vi "5_SPA_KEYSIGHT_rabi_measurements_(SPA_Aver_Mult_traces-Rabi).vi"() -> ()   [LabVIEW 2013]
uses:
  <vilib>/Analysis/baseanly.llb/Mean (DBL).vi
  <vilib>/Analysis/NI_AALBase.lvlib
panel:
  out "x/y":dbl
  out "Normalised":dbl[][](graph)
  out "(Current)":i32=103
  in  "Program to run":u16(ring) items=["Rabi", "T2"]
  in  "?":enum32{"VNA", "SPA"}(tab)
  in  "Center Freq (Hz)":dbl=6953330000.0 caption="Center Freq (Hz):" format="%#.6p"
  in  "VNA Power dBm":dbl=-10.0 caption="VNA Power (dBm)" format="%#.3f"
  in  "Points":i32=2147483647 caption="Center Freq (Hz):"
  in  "Span (Hz)":dbl=6953330000.0 caption="Center Freq (Hz):" format="%#.6p"
  in  "RBW (Hz)":dbl=6953330000.0 caption="Center Freq (Hz):" format="%#.6p"
  in  "VBW (Hz)":dbl=6953330000.0 caption="Center Freq (Hz):" format="%#.6p"
  in  "Averages":u32=251
  out "Background":dbl[][](graph)
  out "Signal":dbl[][](graph)
  out "(Current)":i32=103
  out "Background":dbl[](graph)
  in  "Numeric":u32=251
  in  "Start (ns)":dbl=2.0
  in  "End (ns)":dbl=52.0
  out "Normalised Signal":dbl[][](graph)
  out "Signal":dbl[](graph)
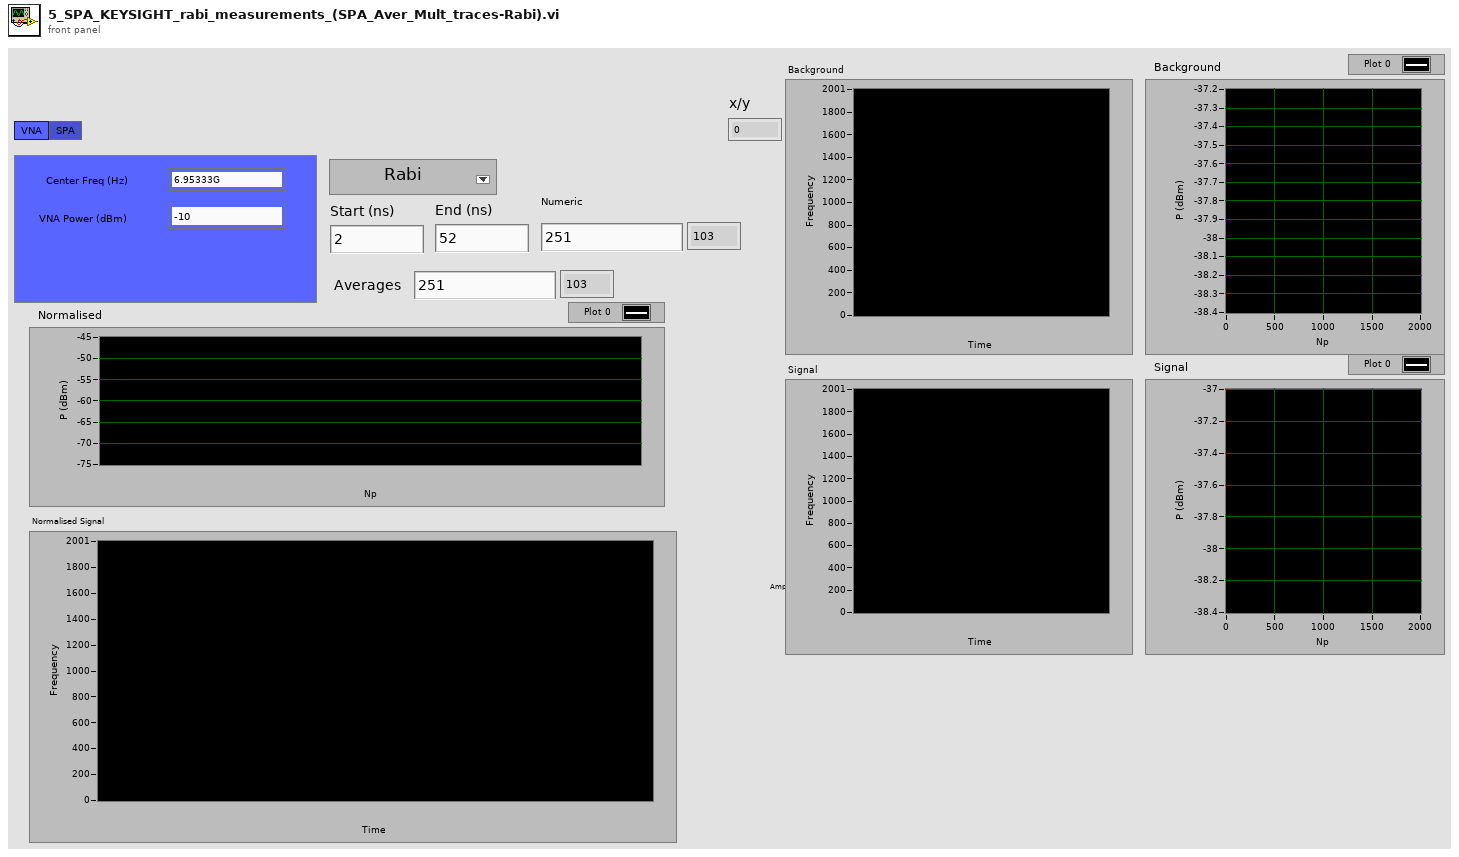
[diagram p1: front panel]
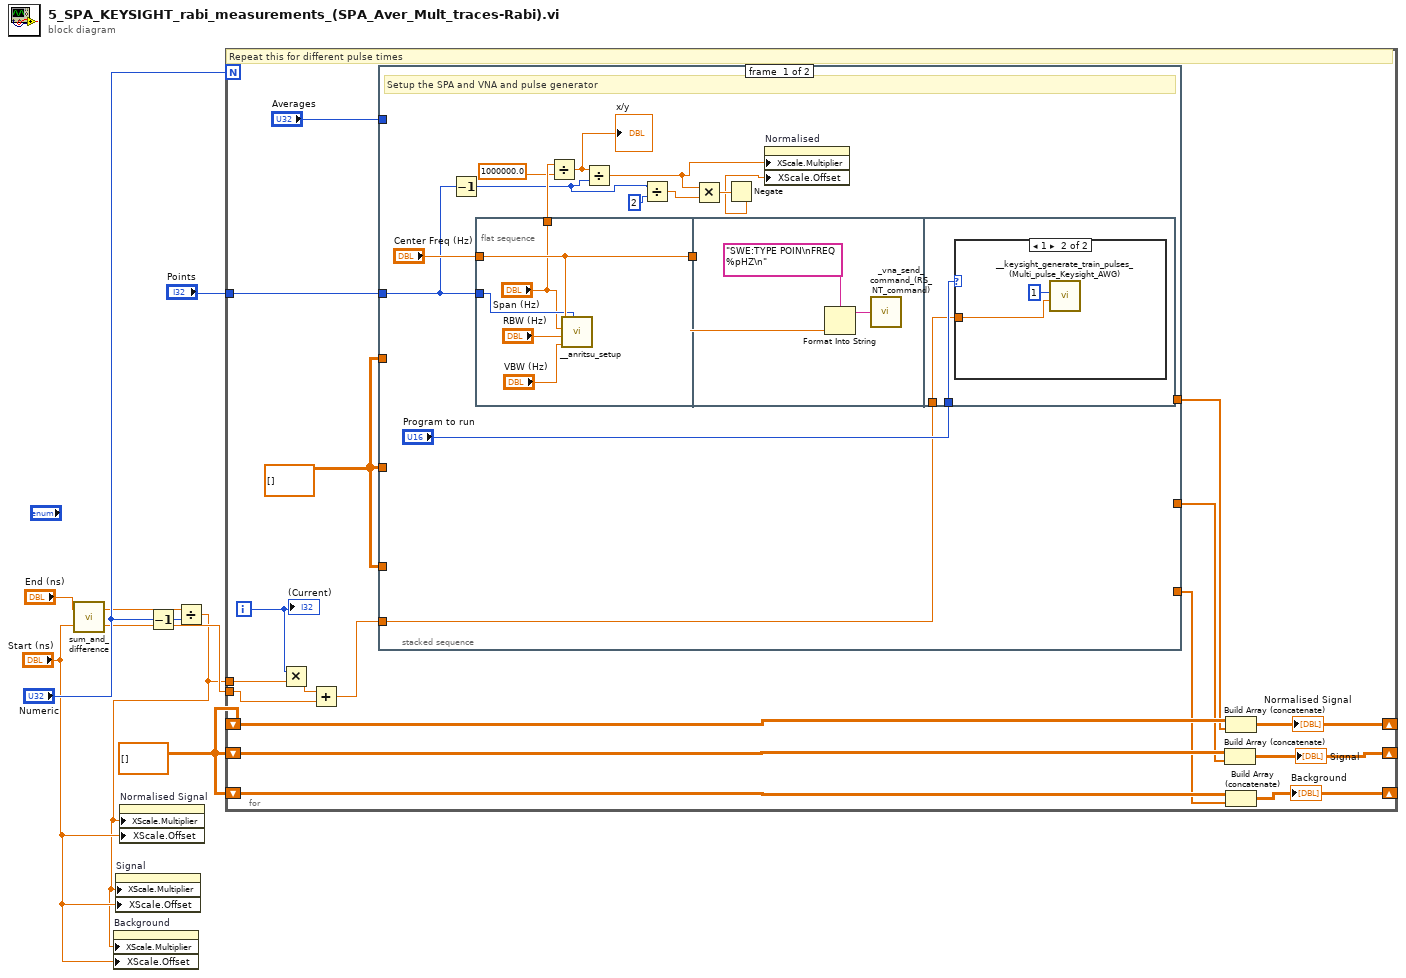
[diagram p0: block diagram]
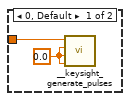
[diagram p2: hidden frame]
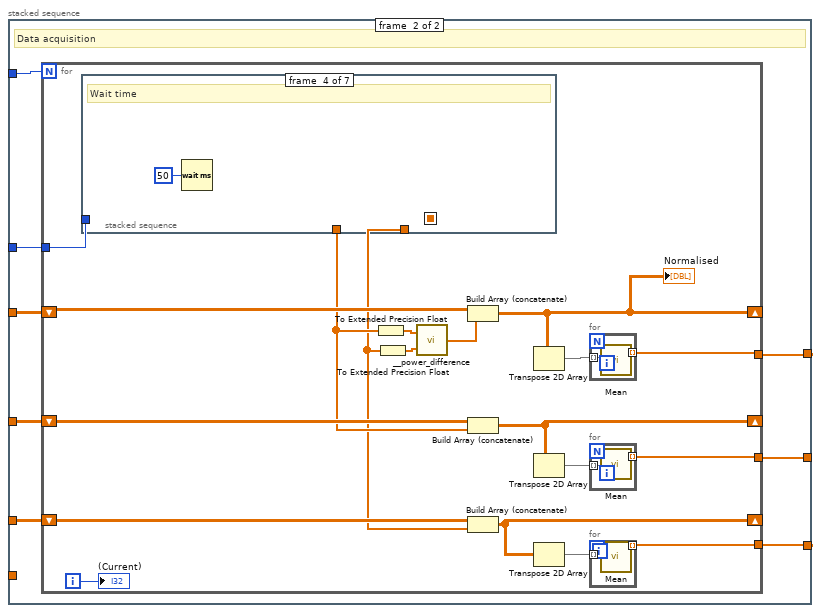
[diagram p3: hidden frame]
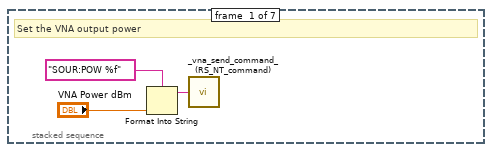
[diagram p4: hidden frame]
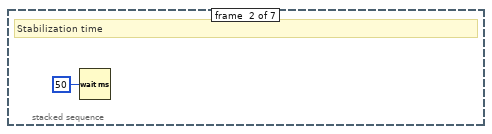
[diagram p5: hidden frame]
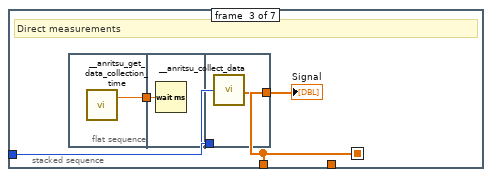
[diagram p6: hidden frame]
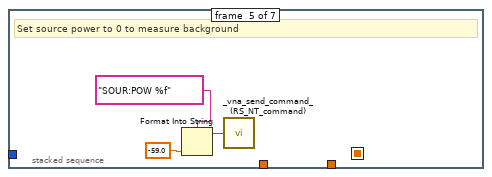
[diagram p7: hidden frame]
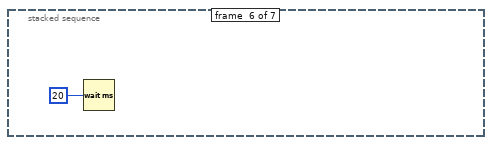
[diagram p8: hidden frame]
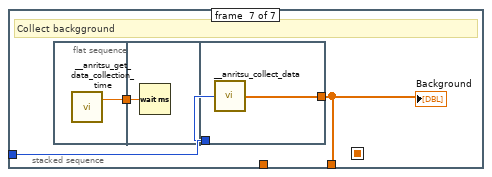
[diagram p9: hidden frame]
diagram:
  w4 = dbl[][] [] ("initialized array")
  n1 = call "sum_and_difference.vi"("Begin"="Start (ns)", "End"="End (ns)") -> ("Difference (abs)"=w5:dbl)  [unwired: 1 out]
  n2 = Decrement(x="Numeric") -> (x-1=w8:u32)
  n3 = Divide(x=w5, y=w8) -> (x/y=w1:dbl)
  n4 = property on="Background" class="IntGraph (strict)"("XScale.Multiplier"=w1, "XScale.Offset"="Start (ns)") -> ()  [unwired: 2 in, 2 out]
  n5 = property on="Signal" class="IntGraph (strict)"("XScale.Multiplier"=w1, "XScale.Offset"="Start (ns)") -> ()  [unwired: 2 in, 2 out]
  n6 = property on="Normalised Signal" class="IntGraph (strict)"("XScale.Multiplier"=w1, "XScale.Offset"="Start (ns)") -> ()  [unwired: 2 in, 2 out]
  n7 = for {
    N: "Numeric" -> [_]
    shift-right: [w22] -> _
    shift-left: w4 -> [w24]
    tunnel: w1 -> [w11]
    tunnel: "Start (ns)" -> [w13]
    shift-right: [w17] -> _
    shift-left: w4 -> [w21]
    shift-right: [w16] -> _
    shift-left: w4 -> [w20]
    tunnel: "Points" -> [w9]
    i -> [w12]
    w15 = dbl[][] [] ("initialized array")
    # "Repeat this for different pulse times"
    n8 = Multiply(x=w12, y=w11) -> (x*y=w10:dbl)
    n9 = Add(x=w10, y=w13) -> (x+y=w14:dbl)
    n10 = stacked-sequence {
      tunnel: "Averages" -> [_ w61]
      tunnel: [_ w60] -> w23
      tunnel: [_ w59] -> w19
      tunnel: [_ w58] -> w18
      tunnel: w15 -> [_ w57]
      tunnel: w15 -> [_ w56]
      tunnel: w15 -> [_ w55]
      tunnel: w14 -> [w37 _]
      tunnel: w9 -> [w27 w54]
      frame #0 {
        # "Setup the SPA and VNA and pulse generator"
        n11 = Decrement(x=w27) -> (x-1=w26:i32)
        n12 = flat-sequence {
          tunnel: w27 -> [w43]
          tunnel: "Center Freq (Hz)" -> [w44]
          tunnel: [w44] -> w39
          tunnel: ["Span (Hz)"] -> w35
          tunnel: w39 -> [w45]
          tunnel: "Program to run" -> [w49]
          tunnel: w37 -> [w48]
          frame #0 {
            n13 = call "__anritsu_setup.vi"("Center Freq (Hz)"=w44, "Span (Hz)"="Span (Hz)", "RBW (Hz)"="RBW (Hz)", "VBW (Hz)"="VBW (Hz)", "Points"=w43) -> ()  [unwired: 1 out]
          }
          frame #1 {
            n14 = Format Into String(format string="SWE:TYPE POIN\nFREQ %pHZ\n" ("Comand"), w45) -> (resulting string=w47:string)  [unwired: 2 in, 1 out]
            n15 = call "_vna_send_command_(RS_NT_command).vi"("Comand"=w47) -> ()  [unwired: 4 in, 1 out]
          }
          frame #2 {
            n16 = case shown="1" w49 {
              tunnel: w48 -> [w50 w52]
              frame 0, Default {
                w51 = 0.0 ("x")
                n17 = call "__keysight_generate_pulses.vi"("Ch1 pulse_width (ns)"=w50, "Ch2 pulse_width (ns)"=w51, "Ch1 pulse_delay (ns)"=w51, "Ch2 pulse_delay (ns)"=w51) -> ()  [unwired: 1 in, 2 out]
              }
              frame 1 {
                n18 = call "__keysight_generate_train_pulses_(Multi_pulse_Keysight_AWG).vi"("start (ns)"=w52, "N"=1) -> ()  [unwired: 10 in]
              }
            }
          }
        }
        n19 = Divide(x=w35, y=1000000.0) -> (x/y=w33:dbl)
        "x/y" <- w33
        n20 = Divide(x=w33, y=w26) -> (x/y=w31:dbl)
        n21 = Divide(x=w26, y=2) -> (x/y=w30:dbl)
        n22 = Multiply(x=w31, y=w30) -> (x*y=w29:dbl)
        n23 = Negate(x=w29) -> (-x=w28:dbl)
        n24 = property on="Normalised" class="WFGraph (strict)"("XScale.Multiplier"=w31, "XScale.Offset"=w28) -> ()  [unwired: 2 in, 2 out]
      }
      frame #1 {
        # "Data acquisition"
        n25 = for {
          N: w61 -> [_]
          shift-right: [w62] -> _
          shift-left: w57 -> [w80]
          tunnel: [w78] -> w60
          shift-right: [w72] -> _
          shift-left: w56 -> [w76]
          shift-right: [w71] -> _
          shift-left: w55 -> [w75]
          tunnel: [w70] -> w59
          tunnel: [w69] -> w58
          tunnel: w54 -> [w68]
          i -> [w77]
          n26 = stacked-sequence {
            seq-local: [_ _ w91 _ _ _ _] -> [_ _ _ _ _ _ _]
            tunnel: [_ _ w91 _ _ _ _] -> w66
            tunnel: [_ _ _ _ _ _ w103] -> w63
            tunnel: w68 -> [_ _ w93 _ _ _ w105]
            frame #0 {
              # "Set the VNA output power"
              n27 = Format Into String(format string="SOUR:POW %f" ("Comand"), "VNA Power dBm") -> (resulting string=w88:string)  [unwired: 2 in, 1 out]
              n28 = call "_vna_send_command_(RS_NT_command).vi"("Comand"=w88) -> ()  [unwired: 4 in, 1 out]
            }
            frame #1 {
              # "Stabilization time"
              n29 = Wait (ms)(milliseconds to wait=u32 50) -> ()  [unwired: 1 out]
            }
            frame #2 {
              # "Direct measurements"
              n30 = flat-sequence {
                tunnel: [w94] -> w92
                tunnel: w92 -> [w95]
                tunnel: [w97] -> w91
                tunnel: w93 -> [w96]
                frame #0 {
                  n31 = call "__anritsu_get_data_collection_time.vi"() -> ("Time to wait (ms)"=w94:dbl)  [unwired: 1 out]
                }
                frame #1 {
                  n32 = Wait (ms)(milliseconds to wait=w95) -> ()  [unwired: 1 out]
                }
                frame #2 {
                  n33 = call "__anritsu_collect_data.vi"("Points to read"=w96) -> ("Data out"=w97:dbl[])
                }
              }
              "Signal" <- w91
            }
            frame #3 {
              # "Wait time"
              n34 = Wait (ms)(milliseconds to wait=u32 50) -> ()  [unwired: 1 out]
            }
            frame #4 {
              # "Set source power to 0 to measure background"
              n35 = Format Into String(format string="SOUR:POW %f" ("Comand"), -59.0 ("input 2")) -> (resulting string=w100:string)  [unwired: 2 in, 1 out]
              n36 = call "_vna_send_command_(RS_NT_command).vi"("Comand"=w100) -> ()  [unwired: 4 in, 1 out]
            }
            frame #5 {
              n37 = Wait (ms)(milliseconds to wait=u32 20) -> ()  [unwired: 1 out]
            }
            frame #6 {
              # "Collect backgground"
              n38 = flat-sequence {
                tunnel: [w106] -> w104
                tunnel: w104 -> [w107]
                tunnel: w105 -> [w109]
                tunnel: [w108] -> w103
                frame #0 {
                  n39 = call "__anritsu_get_data_collection_time.vi"() -> ("Time to wait (ms)"=w106:dbl)  [unwired: 1 out]
                }
                frame #1 {
                  n40 = Wait (ms)(milliseconds to wait=w107) -> ()  [unwired: 1 out]
                }
                frame #2 {
                  n41 = call "__anritsu_collect_data.vi"("Points to read"=w109) -> ("Data out"=w108:dbl[])
                }
              }
              "Background" <- w103
            }
          }
          n42 = To Extended Precision Float(1:w66) -> (0:w65:ext[])
          n43 = To Extended Precision Float(1:w63) -> (0:w64:ext[])
          n44 = call "__power_difference.vi"("Power Low dBm"=w64, "Power High dBm"=w65) -> ("Power Difference dBm"=w67:dbl[])
          n45 = Build Array (concatenate)(w80, w67) -> (w62:dbl[][])
          "Normalised" <- w62
          n46 = Build Array (concatenate)(w76, w66) -> (w72:dbl[][])
          n47 = Build Array (concatenate)(w75, w63) -> (w71:dbl[][])
          n48 = Transpose 2D Array(2D array=w62) -> (transposed array=w79:dbl[][])
          n49 = Transpose 2D Array(2D array=w72) -> (transposed array=w74:dbl[][])
          n50 = Transpose 2D Array(2D array=w71) -> (transposed array=w73:dbl[][])
          n51 = for {
            tunnel: w79 -> [w86] mode=indexing
            tunnel: [w85] -> w78 mode=indexing
            n52 = call-poly <vilib>:"Mean.vi"("X"=w86) -> ("mean"=w85:dbl)  [unwired: 1 out]
          }
          n53 = for {
            tunnel: w74 -> [w84] mode=indexing
            tunnel: [w83] -> w70 mode=indexing
            n54 = call-poly <vilib>:"Mean.vi"("X"=w84) -> ("mean"=w83:dbl)  [unwired: 1 out]
          }
          n55 = for {
            tunnel: w73 -> [w82] mode=indexing
            tunnel: [w81] -> w69 mode=indexing
            n56 = call-poly <vilib>:"Mean.vi"("X"=w82) -> ("mean"=w81:dbl)  [unwired: 1 out]
          }
          "(Current)" <- w77
        }
      }
    }
    n57 = Build Array (concatenate)(w21, w19) -> (w17:dbl[][])
    "Signal" <- w17
    n58 = Build Array (concatenate)(w24, w23) -> (w22:dbl[][])
    "Normalised Signal" <- w22
    n59 = Build Array (concatenate)(w20, w18) -> (w16:dbl[][])
    "Background" <- w16
    "(Current)" <- w12
  }
